vi "Serialize - JSON.vi"(8 "error in":errorcluster, 11 "PAS Data in":refnum<class "PAS Data.lvclass">) -> (0 "error out":errorcluster, 2 "Serialized JSON":string, 3 "PAS Data out":refnum<class "PAS Data.lvclass">)   [LabVIEW 2014, in "PAS Library.lvlib" / "PAS Data.lvclass"]
uses:
  PAS Data.lvclass
  PAS Data.lvclass/PAS Data.ctl
  Cell/PAS Cell Data.lvclass
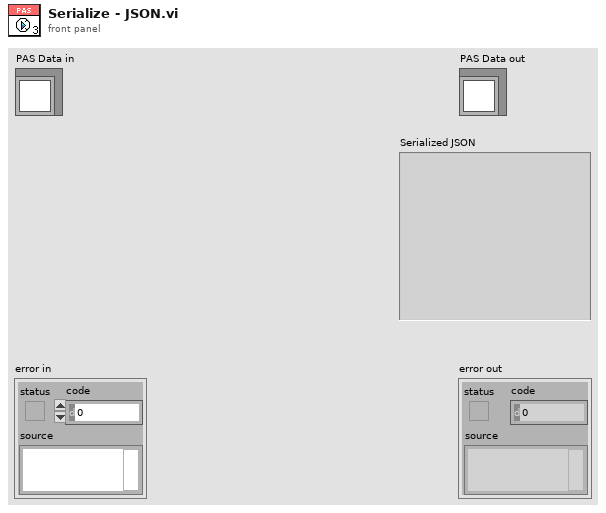
[diagram p1: front panel]
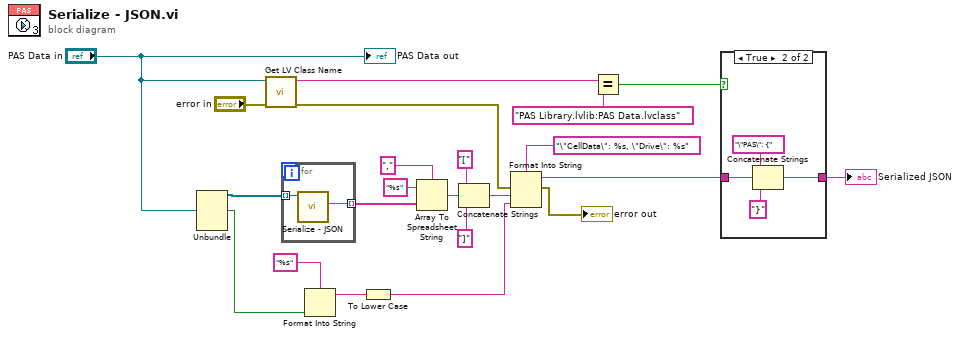
[diagram p0: block diagram]
diagram:
  n1 = Unbundle("PAS Data in") -> (w22:refnum<class "PAS Cell Data.lvclass">[], w4:bool)  [unwired: 3 out]
  n2 = call <vilib>:"Get LV Class Name.vi"("error in (no error)"="error in", "object"="PAS Data in") -> ("error out"=w6:errorcluster, "class name"=w12:string)  [unwired: 8 in]
  n3 = for {
    tunnel: w22 -> [w24] mode=indexing
    tunnel: [w23] -> w21 mode=indexing
    n4 = call-dynamic "Serialize - JSON.vi"("PAS Cell Data in"=w24) -> ("Serialized JSON"=w23:string)  [unwired: 8 in, 2 out]
  }
  n5 = Format Into String(format string="%s", w4) -> (resulting string=w2:string)  [unwired: 2 in, 1 out]
  n6 = To Lower Case(string=w2) -> (all lower case string=w1:string)
  n7 = Array To Spreadsheet String(delimiter (Tab)=",", array=w21, 3:"%s" ("format string")) -> (spreadsheet string=w18:string)
  n8 = Concatenate Strings("[" ("string"), w18, "]" ("string")) -> (w15:string)
  n9 = Format Into String(format string="\"CellData\": %s, \"Drive\": %s", error in=w6, w15, w1) -> (resulting string=w9:string, error out=→"error out":errorcluster)  [unwired: 1 in]
  n10 = Equal?(x=w12, y="PAS Library.lvlib:PAS Data.lvclass") -> (x = y?=w10:bool)
  n11 = case shown="True" w10 {
    tunnel: w9 -> [w25 w29]
    tunnel: [w25 w26] -> w8
    frame False {
    }
    frame True {
      n12 = Concatenate Strings("\"PAS\": {" ("string"), w29, "}" ("string")) -> (w26:string)
    }
  }
  "Serialized JSON" <- w8
  "PAS Data out" <- "PAS Data in"
